vi "CascadeWindows.vi"(8 "error in (no error)":errorcluster, 10 "lpKids":u32[](array[numeric])=[1968530, 4786782, 7866846], 11 "hWnd":u32) -> (0 "error out":errorcluster)   [LabVIEW 2025, in "Test Unit.lvlib"]
uses:
  Test Unit.lvlib
  user32.dll
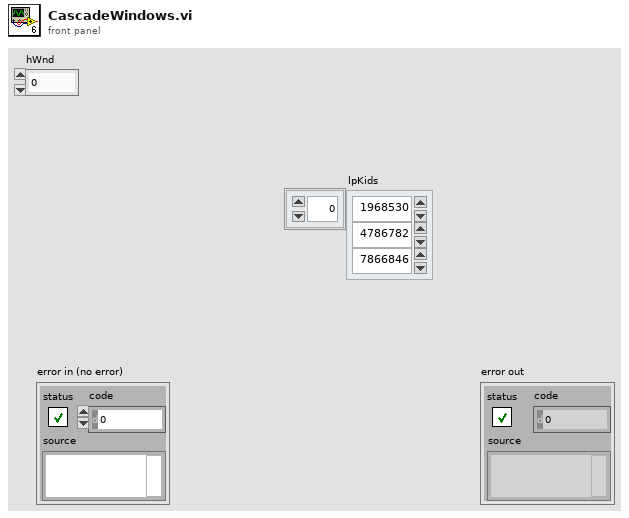
[diagram p1: front panel]
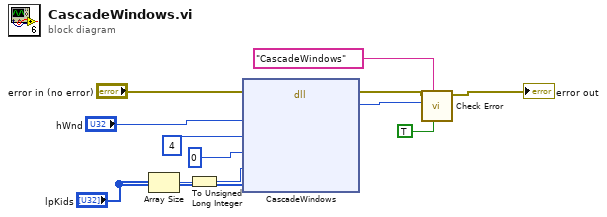
[diagram p0: block diagram]
diagram:
  n1 = Array Size(array="lpKids") -> (size(s)=w4:i32)
  n2 = To Unsigned Long Integer(number=w4) -> (unsigned 32bit integer=w1:u32)
  n3 = dll-call lib="user32.dll" fn="CascadeWindows"(error in="error in (no error)", "hwndParent"="hWnd", "wHow"=u32 4, "rect"=u32 0, "cKids"=w1, "lpKids"="lpKids") -> (error out=w7:errorcluster, "error"=w8:u32)  [unwired: 7 in, 1 out]
  n4 = call "Check Error.vi"("Error on Zero? (f)"=TRUE, "Description"="CascadeWindows" ("Error Action"), "Return Code"=w8, "error in (no error)"=w7) -> ("error out"=→"error out":errorcluster)  [unwired: 7 in]
